vi "Next Environment.vi"(8 "error in (no error)":errorcluster, 11 "Test Framework in":refnum<class "Test Framework.lvclass">) -> (0 "error out":errorcluster, 2 "User canceled":bool, 3 "Test Framework out":refnum<class "Test Framework.lvclass">)   [LabVIEW 2020, in "Test Framework.lvclass"]
uses:
  Test Framework.lvclass
  Test Framework.lvclass/Test Framework.ctl
  XML Handler/XML Handler.lvclass
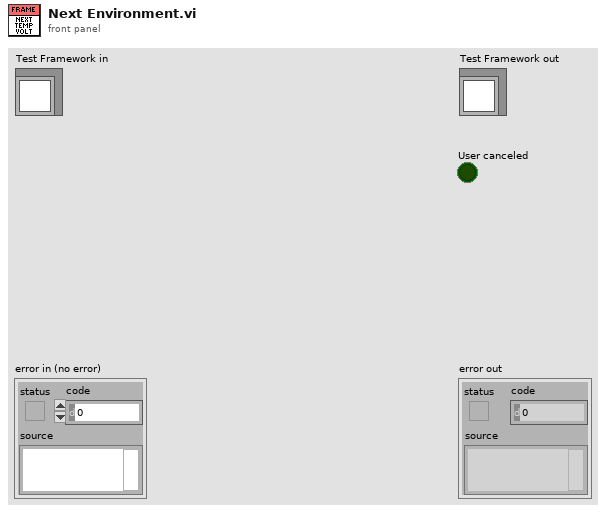
[diagram p1: front panel]
types:
  T1 = cluster{"Temperature [degC]":dbl, "Soak time [s]":dbl, "PSUs":cluster{"PSU alias":string, "Source":enum32{"Voltage", "Current"}, "Drive (V/A)":dbl}[]}
  T2 = typedef "Test Framework.lvclass/Temperature and voltage array.ctl" = cluster{"Temperature [C]":dbl, "Soak time [m]":dbl, "PSUs":cluster{"Enabled":bool, "Source":enum32{"Voltage", "Current"}, "Drive (V/A)":dbl, "Sweep (V/A)":string, "Limit (A/V)":dbl, "PSU alias":string, "PSU info":cluster{"ID":string, "Address":string, "Channel":u8}}[]}[]
  T3 = typedef "Test Framework.lvclass/Temperature and voltage modes.ctl" = cluster{"Temperature mode":enum16{"Automatic", "Manual", "Off"}, "DC-Power mode":enum16{"Automatic", "Manual", "Off"}, "PSU sweep mode":bool, "Turn off after measurement":bool}
  T4 = cluster{"Temperature control array":T2, "Temperature mode":T3}
  T5 = cluster{"Temperature [C]":dbl, "Soak time [m]":dbl, "PSUs":cluster{"Enabled":bool, "Source":enum32{"Voltage", "Current"}, "Drive (V/A)":dbl, "Sweep (V/A)":string, "Limit (A/V)":dbl, "PSU alias":string, "PSU info":cluster{"ID":string, "Address":string, "Channel":u8}}[]}
  T6 = cluster{"PSU alias":string, "Source":enum32{"Voltage", "Current"}, "Drive (V/A)":dbl}[]
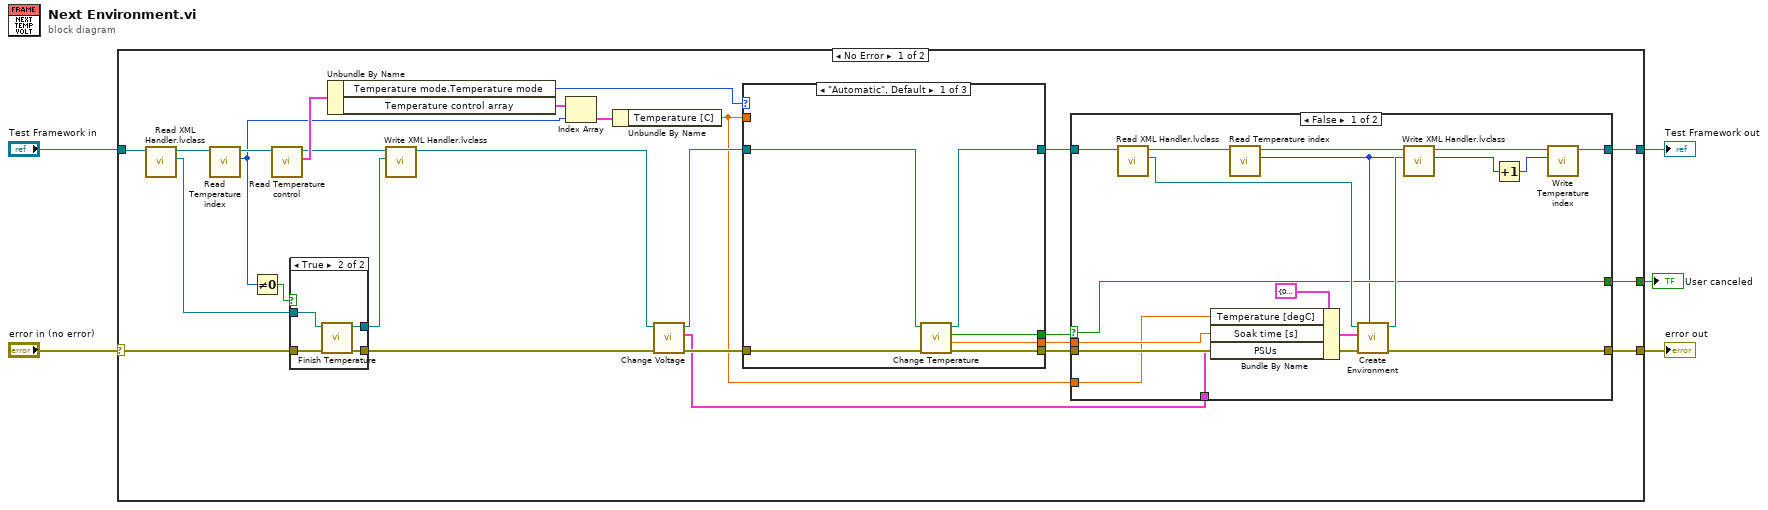
[diagram p0: block diagram]
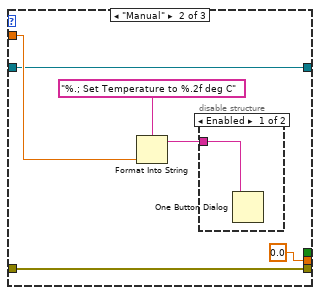
[diagram p3: hidden frame]
diagram:
  n1 = case shown="No Error" "error in (no error)" {
    selector: "error in (no error)" -> [w23 w74]
    tunnel: [w26 w74] -> w4
    tunnel: [w27 w73] -> w2
    tunnel: "Test Framework in" -> [w22 w73]
    tunnel: [w25 _] -> w1
    frame No Error {
      n2 = call "Read XML Handler.lvclass.vi"("Test Framework in"=w22) -> ("XML Handler.lvclass"=w20:refnum<class "XML Handler.lvclass">, "Test Framework out"=w21:refnum<class "Test Framework.lvclass">)  [unwired: 9 in]
      n3 = call "Read Temperature index.vi"("Test Framework in"=w21) -> ("Environmental index"=w8:i32, "Test Framework out"=w18:refnum<class "Test Framework.lvclass">)  [unwired: 9 in]
      n4 = Not Equal To 0?(x=w8) -> (x != 0?=w24:bool)
      n5 = call-dynamic "Read Temperature control.vi"("Test Framework in"=w18) -> ("Temperature control"=w17:T4, "Test Framework out"=w11:refnum<class "Test Framework.lvclass">)  [unwired: 9 in]
      n6 = case shown="True" w24 {
        tunnel: w23 -> [w33 w37]
        tunnel: w20 -> [w32 w36]
        tunnel: [w32 w35] -> w19
        tunnel: [w33 w34] -> w15
        frame False {
        }
        frame True {
          n7 = call "Finish Temperature.vi"("error in (no error)"=w37, "XML Handler in"=w36) -> ("error out"=w34:errorcluster, "XML Handler out"=w35:refnum<class "XML Handler.lvclass">)  [unwired: 8 in]
        }
      }
      n8 = Unbundle By Name(w17) -> ("Temperature mode.Temperature mode"=w16:enum16{"Automatic", "Manual", "Off"}, "Temperature control array"=w9:T2)
      n9 = call "Write XML Handler.lvclass.vi"("XML Handler.lvclass"=w19, "Test Framework in"=w11) -> ("Test Framework out"=w10:refnum<class "Test Framework.lvclass">)  [unwired: 9 in]
      n10 = Index Array(array=w9, index=w8) -> (element=w7:T5)
      n11 = Unbundle By Name(w7) -> ("Temperature [C]"=w6:dbl)
      n12 = call "Change Voltage.vi"("error in (no error)"=w15, "Test Framework in"=w10) -> ("error out"=w14:errorcluster, "PSU status"=w13:T6, "Test Framework out"=w12:refnum<class "Test Framework.lvclass">)  [unwired: 7 in]
      n13 = case shown="\"Automatic\", Default" w16 {
        tunnel: [w43 w48 w51] -> w31
        tunnel: [w42 0.0 ("Soak Time Used") _] -> w30
        tunnel: w12 -> [w41 w44 w52]
        tunnel: [w40 w44 w52] -> w29
        tunnel: [w39 _ _] -> w28
        tunnel: w14 -> [w38 w48 w51]
        tunnel: w6 -> [_ w46 _]
        frame "Automatic", Default {
          n14 = call "Change Temperature.vi"("error in (no error)"=w38, "Test Framework in"=w41) -> ("error out"=w43:errorcluster, "Soak Time Used"=w42:dbl, "User Aborted"=w39:bool, "Test Framework out"=w40:refnum<class "Test Framework.lvclass">)  [unwired: 6 in]
        }
        frame "Manual" {
          n15 = Format Into String(format string="%.; Set Temperature to %.2f deg C", w46) -> (resulting string=w45:string)  [unwired: 2 in, 1 out]
          n16 = disable-structure shown="Enabled" {
            disable-tunnel: w45 -> [w50 _]
            frame Enabled {
              n17 = One Button Dialog(message=w50) -> ()  [unwired: 1 in, 1 out]
            }
            frame Disabled {
            }
          }
        }
        frame "Off" {
        }
      }
      n18 = case shown="False" w28 {
        selector: w28 -> [w61 w70]
        tunnel: w31 -> [w69 w72]
        tunnel: w30 -> [w66 _]
        tunnel: w29 -> [w65 w71]
        tunnel: [w60 w71] -> w27
        tunnel: [w62 w72] -> w26
        tunnel: [w61 w70] -> w25
        tunnel: w13 -> [w58 _]
        tunnel: w6 -> [w57 _]
        frame False {
          n19 = call "Read XML Handler.lvclass.vi"("Test Framework in"=w65) -> ("XML Handler.lvclass"=w68:refnum<class "XML Handler.lvclass">, "Test Framework out"=w56:refnum<class "Test Framework.lvclass">)  [unwired: 9 in]
          n20 = Bundle By Name(cluster=T1 {"Temperature [degC]"=0.0, "Soak time [s]"=0.0, "PSUs"=[]} ("Temperature info"), "Temperature [degC]"=w57, "Soak time [s]"=w66, "PSUs"=w58) -> (w64:T1)
          n21 = call "Read Temperature index.vi"("Test Framework in"=w56) -> ("Environmental index"=w53:i32, "Test Framework out"=w55:refnum<class "Test Framework.lvclass">)  [unwired: 9 in]
          n22 = call "Create Environment.vi"("Environmental index"=w53, "error in (no error)"=w69, "Environmental info"=w64, "XML Handler in"=w68) -> ("error out"=w62:errorcluster, "XML Handler out"=w63:refnum<class "XML Handler.lvclass">)  [unwired: 6 in]
          n23 = call "Write XML Handler.lvclass.vi"("XML Handler.lvclass"=w63, "Test Framework in"=w55) -> ("Test Framework out"=w54:refnum<class "Test Framework.lvclass">)  [unwired: 9 in]
          n24 = Increment(x=w53) -> (x+1=w59:i32)
          n25 = call "Write Temperature index.vi"("Environmental index"=w59, "Test Framework in"=w54) -> ("Test Framework out"=w60:refnum<class "Test Framework.lvclass">)  [unwired: 9 in]
        }
        frame True {
        }
      }
    }
    frame Error {
    }
  }
  "error out" <- w4
  "Test Framework out" <- w2
  "User canceled" <- w1
